vi "ReadData.vi"(8 "error in":errorcluster, 11 "Module Config Selector":i16) -> (0 "error out":errorcluster, 3 "Data Array":sgl[](array[numeric]) format="%.2f")   [LabVIEW 2017, in "BOP_VibAPI_6.lvlib"]
uses:
  <vilib>/addons/InsightCM/Devices/Shared/Cms/Fpga/Acquisition/source/subVIs/VibAPI/BOP_VibAPI_6.lvlib
  <vilib>/eio/EIONode/EIONode.xnode
  <vilib>/rvi/eio/common/nirviEmuTemplateMethod_errors.vi
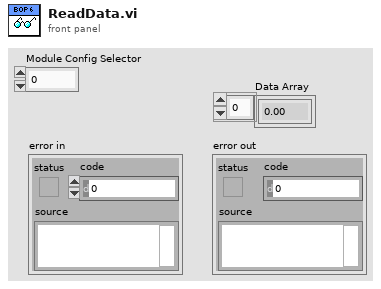
[diagram p1: front panel]
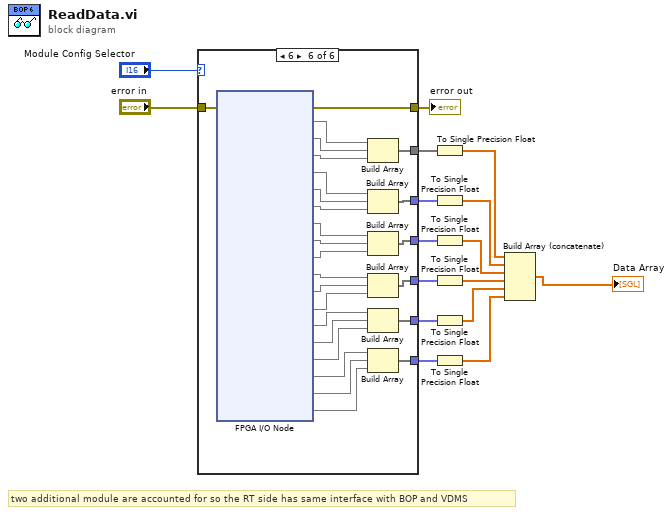
[diagram p0: block diagram]
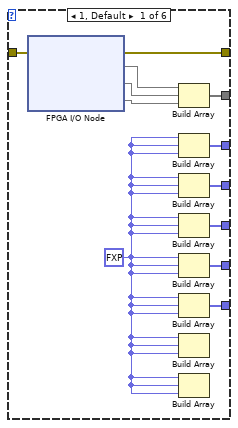
[diagram p2: hidden frame]
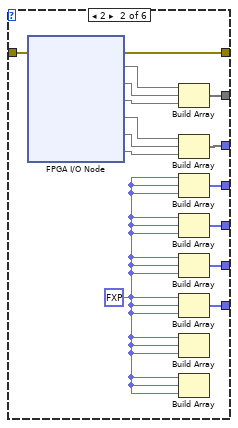
[diagram p3: hidden frame]
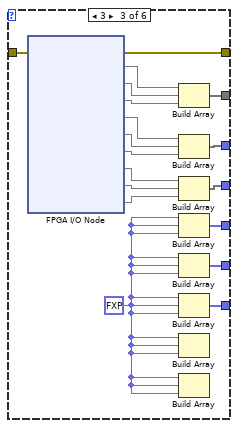
[diagram p4: hidden frame]
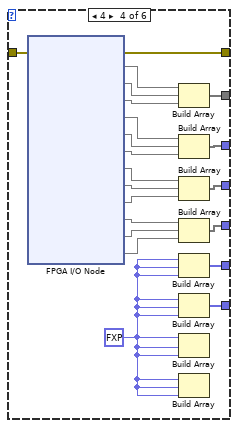
[diagram p5: hidden frame]
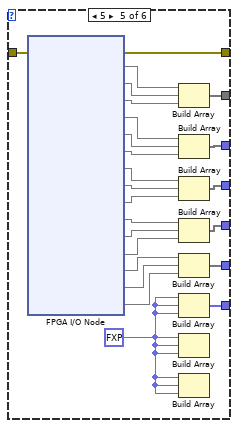
[diagram p6: hidden frame]
diagram:
  # "two additional module are accounted for so the RT side has same interface with BOP and VDMS"
  n1 = case shown="6" "Module Config Selector" {
    tunnel: "error in" -> [w25 w40 w58 w79 w103 w129]
    tunnel: [w24 w39 w57 w78 w102 w128] -> w15
    tunnel: [w23 w38 w56 w77 w101 w127] -> w13
    tunnel: [w22 w37 w55 w76 w100 w126] -> w10
    tunnel: [w21 w36 w54 w75 w99 w125] -> w9
    tunnel: [w20 w35 w53 w74 w98 w124] -> w8
    tunnel: [w19 w34 w52 w73 w97 w123] -> w7
    tunnel: [w18 w33 w51 w72 w96 w122] -> w6
    frame 1, Default {
      w17 = fxp<+/-,24,7> 0.0 ("Mod1/AI2")
      n2 = xnode "FPGA I/O Node"("error in"=w25) -> ("error out"=w24:errorcluster, "Mod1/AI0"=w26, "Mod1/AI1"=w28, "Mod1/AI2"=w27)  [unwired: 3 in, 3 out]
      n3 = Build Array(w26, w28, w27) -> (w23:void[])
      n4 = Build Array(w17, w17, w17) -> (w22:fxp<+/-,24,7>[])
      n5 = Build Array(w17, w17, w17) -> (w21:fxp<+/-,24,7>[])
      n6 = Build Array(w17, w17, w17) -> (w20:fxp<+/-,24,7>[])
      n7 = Build Array(w17, w17, w17) -> (w19:fxp<+/-,24,7>[])
      n8 = Build Array(w17, w17, w17) -> (w18:fxp<+/-,24,7>[])
      n9 = Build Array(w17, w17, w17) -> ()  [unwired: 1 out]
      n10 = Build Array(w17, w17, w17) -> ()  [unwired: 1 out]
    }
    frame 2 {
      w29 = fxp<+/-,24,7> 0.0 ("Mod1/AI2")
      n11 = xnode "FPGA I/O Node"("error in"=w40) -> ("error out"=w39:errorcluster, "Mod1/AI0"=w41, "Mod1/AI1"=w43, "Mod1/AI2"=w42, "Mod2/AI0"=w32, "Mod2/AI1"=w31, "Mod2/AI2"=w30)  [unwired: 6 in, 6 out]
      n12 = Build Array(w41, w43, w42) -> (w38:void[])
      n13 = Build Array(w32, w31, w30) -> (w37:void[])
      n14 = Build Array(w29, w29, w29) -> (w36:fxp<+/-,24,7>[])
      n15 = Build Array(w29, w29, w29) -> (w35:fxp<+/-,24,7>[])
      n16 = Build Array(w29, w29, w29) -> (w34:fxp<+/-,24,7>[])
      n17 = Build Array(w29, w29, w29) -> (w33:fxp<+/-,24,7>[])
      n18 = Build Array(w29, w29, w29) -> ()  [unwired: 1 out]
      n19 = Build Array(w29, w29, w29) -> ()  [unwired: 1 out]
    }
    frame 3 {
      w44 = fxp<+/-,24,7> 0.0 ("Mod1/AI2")
      n20 = xnode "FPGA I/O Node"("error in"=w58) -> ("error out"=w57:errorcluster, "Mod1/AI0"=w59, "Mod1/AI1"=w61, "Mod1/AI2"=w60, "Mod2/AI0"=w50, "Mod2/AI1"=w49, "Mod2/AI2"=w48, "Mod3/AI0"=w47, "Mod3/AI1"=w46, "Mod3/AI2"=w45)  [unwired: 9 in, 9 out]
      n21 = Build Array(w59, w61, w60) -> (w56:void[])
      n22 = Build Array(w50, w49, w48) -> (w55:void[])
      n23 = Build Array(w47, w46, w45) -> (w54:void[])
      n24 = Build Array(w44, w44, w44) -> (w53:fxp<+/-,24,7>[])
      n25 = Build Array(w44, w44, w44) -> (w52:fxp<+/-,24,7>[])
      n26 = Build Array(w44, w44, w44) -> (w51:fxp<+/-,24,7>[])
      n27 = Build Array(w44, w44, w44) -> ()  [unwired: 1 out]
      n28 = Build Array(w44, w44, w44) -> ()  [unwired: 1 out]
    }
    frame 4 {
      w62 = fxp<+/-,24,7> 0.0 ("Mod1/AI2")
      n29 = xnode "FPGA I/O Node"("error in"=w79) -> ("error out"=w78:errorcluster, "Mod1/AI0"=w80, "Mod1/AI1"=w82, "Mod1/AI2"=w81, "Mod2/AI0"=w71, "Mod2/AI1"=w70, "Mod2/AI2"=w69, "Mod3/AI0"=w68, "Mod3/AI1"=w67, "Mod3/AI2"=w66, "Mod4/AI0"=w65, "Mod4/AI1"=w64, "Mod4/AI2"=w63)  [unwired: 12 in, 12 out]
      n30 = Build Array(w80, w82, w81) -> (w77:void[])
      n31 = Build Array(w71, w70, w69) -> (w76:void[])
      n32 = Build Array(w68, w67, w66) -> (w75:void[])
      n33 = Build Array(w65, w64, w63) -> (w74:void[])
      n34 = Build Array(w62, w62, w62) -> (w73:fxp<+/-,24,7>[])
      n35 = Build Array(w62, w62, w62) -> (w72:fxp<+/-,24,7>[])
      n36 = Build Array(w62, w62, w62) -> ()  [unwired: 1 out]
      n37 = Build Array(w62, w62, w62) -> ()  [unwired: 1 out]
    }
    frame 5 {
      w83 = fxp<+/-,24,7> 0.0 ("Mod1/AI2")
      n38 = xnode "FPGA I/O Node"("error in"=w103) -> ("error out"=w102:errorcluster, "Mod1/AI0"=w104, "Mod1/AI1"=w106, "Mod1/AI2"=w105, "Mod2/AI0"=w95, "Mod2/AI1"=w94, "Mod2/AI2"=w93, "Mod3/AI0"=w92, "Mod3/AI1"=w91, "Mod3/AI2"=w90, "Mod4/AI0"=w89, "Mod4/AI1"=w88, "Mod4/AI2"=w87, "Mod5/AI0"=w86, "Mod5/AI1"=w85, "Mod5/AI2"=w84)  [unwired: 15 in, 15 out]
      n39 = Build Array(w104, w106, w105) -> (w101:void[])
      n40 = Build Array(w95, w94, w93) -> (w100:void[])
      n41 = Build Array(w92, w91, w90) -> (w99:void[])
      n42 = Build Array(w89, w88, w87) -> (w98:void[])
      n43 = Build Array(w86, w85, w84) -> (w97:void[])
      n44 = Build Array(w83, w83, w83) -> (w96:fxp<+/-,24,7>[])
      n45 = Build Array(w83, w83, w83) -> ()  [unwired: 1 out]
      n46 = Build Array(w83, w83, w83) -> ()  [unwired: 1 out]
    }
    frame 6 {
      n47 = xnode "FPGA I/O Node"("error in"=w129) -> ("error out"=w128:errorcluster, "Mod1/AI0"=w130, "Mod1/AI1"=w132, "Mod1/AI2"=w131, "Mod2/AI0"=w121, "Mod2/AI1"=w120, "Mod2/AI2"=w119, "Mod3/AI0"=w118, "Mod3/AI1"=w117, "Mod3/AI2"=w116, "Mod4/AI0"=w115, "Mod4/AI1"=w114, "Mod4/AI2"=w113, "Mod5/AI0"=w112, "Mod5/AI1"=w111, "Mod5/AI2"=w110, "Mod6/AI0"=w109, "Mod6/AI1"=w108, "Mod6/AI2"=w107)  [unwired: 18 in, 18 out]
      n48 = Build Array(w130, w132, w131) -> (w127:void[])
      n49 = Build Array(w121, w120, w119) -> (w126:void[])
      n50 = Build Array(w118, w117, w116) -> (w125:void[])
      n51 = Build Array(w115, w114, w113) -> (w124:void[])
      n52 = Build Array(w112, w111, w110) -> (w123:void[])
      n53 = Build Array(w109, w108, w107) -> (w122:void[])
    }
  }
  "error out" <- w15
  n54 = To Single Precision Float(number=w13) -> (single precision float=w12:sgl[])
  n55 = To Single Precision Float(number=w10) -> (single precision float=w5:sgl[])
  n56 = To Single Precision Float(number=w9) -> (single precision float=w4:sgl[])
  n57 = To Single Precision Float(number=w8) -> (single precision float=w3:sgl[])
  n58 = To Single Precision Float(number=w7) -> (single precision float=w2:sgl[])
  n59 = To Single Precision Float(number=w6) -> (single precision float=w1:sgl[])
  n60 = Build Array (concatenate)(w12, w5, w4, w3, w2, w1) -> (→"Data Array":sgl[])
